vi "REx - Send Command Core.vi"(0 "LVx Command in":refnum<class "LVx.lvclass">, 1 "port number(3363)":u16=3363, 2 "machine name (LocalApp:\"\")":string, 11 "error in (no error)":errorcluster, 12 "Retain Session (F)":bool, 13 "Session ID":string) -> (4 "LVx Command response":refnum<class "LVx.lvclass">, 15 "error out":errorcluster)   [LabVIEW 2011, in "LVx.lvlib" / "LVx.lvclass"]
uses:
  LVx.lvclass
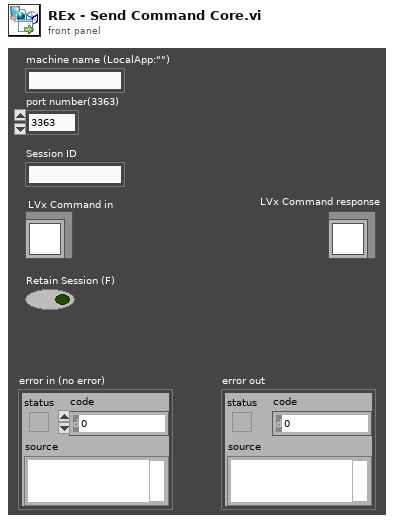
[diagram p1: front panel]
types:
  T1 = cluster{"machine name (LocalApp:\"\")":string, "port number(3363)":u16}
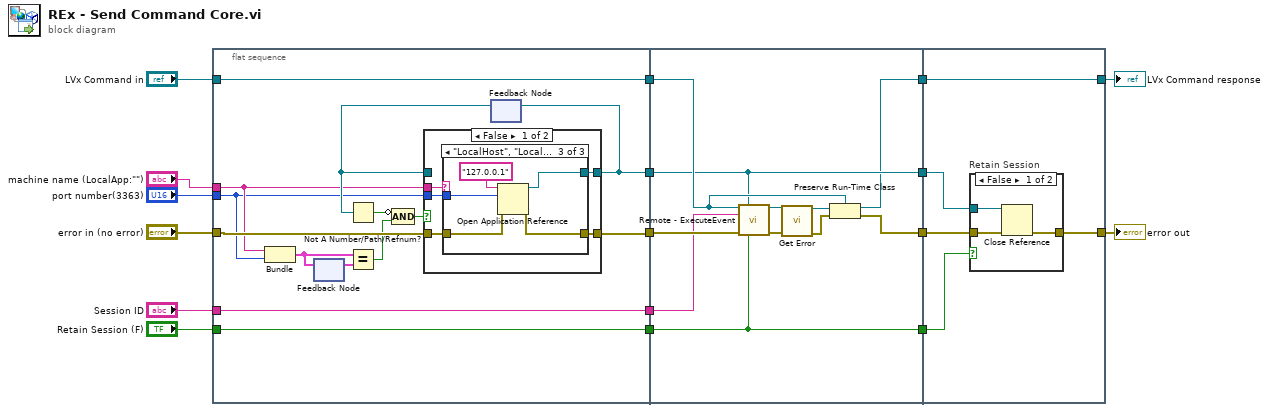
[diagram p0: block diagram]
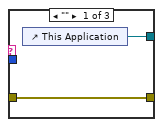
[diagram p2: hidden frame]
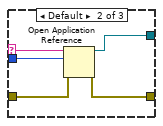
[diagram p3: hidden frame]
diagram:
  n1 = flat-sequence {
    tunnel: "LVx Command in" -> [w28]
    tunnel: "error in (no error)" -> [w30]
    tunnel: "Retain Session (F)" -> [w31]
    tunnel: [w31] -> w11
    tunnel: [w29] -> w10
    tunnel: "port number(3363)" -> [w23]
    tunnel: "machine name (LocalApp:\"\")" -> [w24]
    tunnel: [w26] -> w9
    tunnel: [w28] -> w8
    tunnel: [w27] -> w3
    tunnel: "Session ID" -> [w27]
    tunnel: w11 -> [w55]
    tunnel: w10 -> [w58]
    tunnel: [w59] -> w7
    tunnel: w9 -> [w60]
    tunnel: [w60] -> w6
    tunnel: w8 -> [w61]
    tunnel: [w57] -> w5
    tunnel: w3 -> [w56]
    tunnel: [w55] -> w1
    tunnel: [w65] -> w16
    tunnel: w7 -> [w66]
    tunnel: w6 -> [w63]
    tunnel: [w64] -> w17
    tunnel: w5 -> [w64]
    tunnel: w1 -> [w62]
    frame #0 {
      n2 = Bundle("machine name (LocalApp:\"\")"=w24, "port number(3363)"=w23) -> (w18:T1)  [unwired: 1 in]
      n3 = feedback-in #1(w18) -> ()
      n4 = feedback #1() -> (w19:T1)  [unwired: 1 in]
      n5 = Equal?(x=w18, y=w19) -> (x = y?=w21:bool)
      n6 = feedback #2() -> (w25:refnum<vi>)  [unwired: 1 in]
      n7 = Not A Number/Path/Refnum?(number/path/refnum=w25) -> (NaN/Path/Refnum?=w22:bool)
      n8 = Compound Arithmetic op=AND(invert w22, w21) -> (w20:bool)
      n9 = case shown="False" w20 {
        tunnel: w23 -> [w36 _]
        tunnel: w30 -> [w35 w49]
        tunnel: [w34 w49] -> w29
        tunnel: w24 -> [w33 _]
        tunnel: [w32 w50] -> w26
        tunnel: w25 -> [_ w50]
        frame False {
          n10 = case shown="\"LocalHost\", \"Localhost\", \"localhost\"" w33 {
            selector: w33 -> [_ w42 _]
            tunnel: [w38 w43 w48] -> w32
            tunnel: [w37 w40 w46] -> w34
            tunnel: w35 -> [w37 w39 w44]
            tunnel: w36 -> [_ w41 w47]
            frame "" {
              n11 = control-ref of="This Application"() -> (w38:refnum<vi>)
            }
            frame Default {
              n12 = Open Application Reference(8:w39, 10:w41, 11:w42) -> (0:w40:errorcluster, 3:w43:refnum<vi>)  [unwired: 1 out]
            }
            frame "LocalHost", "Localhost", "localhost" {
              n13 = Open Application Reference(8:w44, 10:w47, 11:"127.0.0.1" ("machine name (Local:\"\")")) -> (0:w46:errorcluster, 3:w48:refnum<vi>)  [unwired: 1 out]
            }
          }
        }
        frame True {
        }
      }
      n14 = feedback-in #2(w26) -> ()
    }
    frame #1 {
      n15 = call "Remote - ExecuteEvent.vi"("LVx Command in"=w61, "application reference"=w60, "Session ID"=w56, "error in (no error)"=w58, "Retain Session (F)"=w55) -> ("LVx Command out"=w54:refnum<class "LVx.lvclass">, "error out"=w53:errorcluster)  [unwired: 9 out]
      n16 = call "Get Error.vi"("LVx.lvlib:LVx.lvclass"=w54, "error in (no error)"=w53) -> ("LVx.lvlib:LVx.lvclass 2"=w52:refnum<class "LVx.lvclass">, "error out"=w51:errorcluster)  [unwired: 12 in]
      n17 = Preserve Run-Time Class(object in=w52, error in=w51, 2:w61) -> (object out=w57:refnum<class "LVx.lvclass">, error out=w59:errorcluster)
    }
    frame #2 {
      n18 = case "Retain Session" shown="False" w62 {
        tunnel: w66 -> [w69 w70]
        tunnel: [w68 w70] -> w65
        tunnel: w63 -> [w67 _]
        frame False {
          n19 = Close Reference(reference=w67, error in (no error)=w69) -> (error out=w68:errorcluster)
        }
        frame True {
        }
      }
    }
  }
  "LVx Command response" <- w17
  "error out" <- w16
